vi "Prepare Response.vi"(8 "error in (no error)":errorcluster, 11 "PUBREL in":refnum<class "PUBREL.lvclass">) -> (0 "error out":errorcluster, 1 "response prepared?":bool, 2 "ControlPacket response":refnum<class "ControlPacket.lvclass">, 3 "PUBREL out":refnum<class "PUBREL.lvclass">)   [LabVIEW 2013, in "MQTT_Control_Packets.lvlib" / "PUBREL.lvclass"]
uses:
  PUBREL.lvclass
  ControlPacket/ControlPacket.lvclass
  ControlPacket/ControlPacket.lvclass/ControlPacket.ctl
  PUBCOMP/PUBCOMP.lvclass
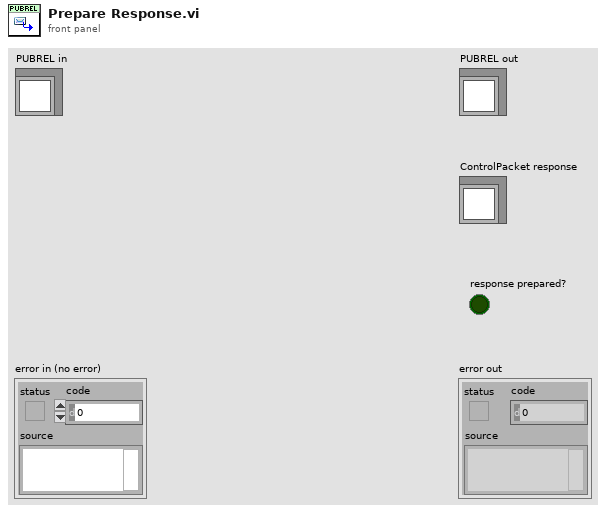
[diagram p1: front panel]
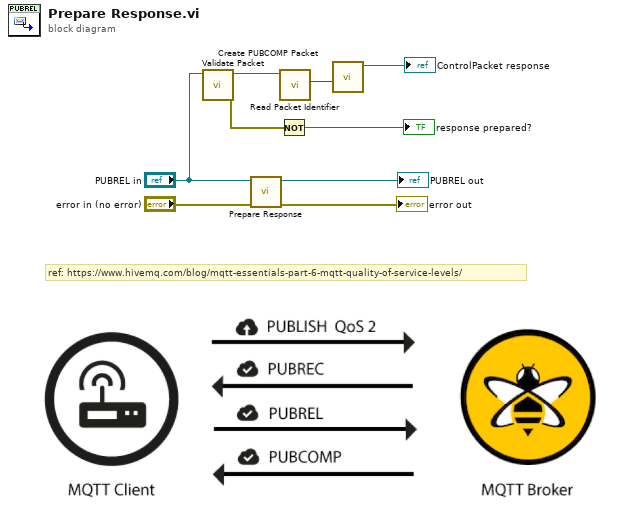
[diagram p0: block diagram]
diagram:
  # "ref: https://www.hivemq.com/blog/mqtt-essentials-part-6-mqtt-quality-of-service-levels/"
  n1 = call "Validate Packet.vi"("ControlPacket in"="PUBREL in") -> ("error out"=w5:errorcluster, "ControlPacket out"=w6:refnum<class "PUBREL.lvclass">)  [unwired: 9 in]
  n2 = call-parent "Prepare Response.vi"("error in (no error)"="error in (no error)", "ControlPacket in"="PUBREL in") -> ("error out"=→"error out":errorcluster, "ControlPacket out"=→"PUBREL out":refnum<class "PUBREL.lvclass">)  [unwired: 6 in, 2 out]
  n3 = Not(x=w5) -> (.not. x?=→"response prepared?":bool)
  n4 = call "Read Packet Identifier.vi"("ControlPacket in"=w6) -> ("Packet Identifier"=w4:u16)  [unwired: 9 in, 1 out]
  n5 = call "Create PUBCOMP Packet.vi"("Packet ID"=w4) -> ("PUBCOMP out"=→"ControlPacket response":refnum<class "PUBCOMP.lvclass">)  [unwired: 9 in, 1 out]
